vi "TextGetTranslatorCount.vi"() -> (8 "Number Of Translations":i32)   [LabVIEW 2011]
uses:
  HelperVIsforTextTranslator.llb/Textarrayglobal.vi
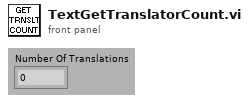
[diagram p1: front panel]
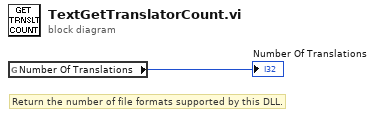
[diagram p0: block diagram]
diagram:
  # "Return the number of file formats supported by this DLL."
  n1 = global read "Textarrayglobal.vi" "Number Of Translations"() -> (→"Number Of Translations":i32)
